vi "Process ILC Data.vi"(8 "error in (no error)":errorcluster, 11 "Model in":refnum<class "Model.lvclass">) -> (0 "error out":errorcluster, 3 "Model out":refnum<class "Model.lvclass">)   [LabVIEW 2016]
uses:
  Common_RT_FAILC/FAILC/FAILC.lvclass
  Calculators/Cylinder To Actuator Forces/Cylinder To Actuator Forces.lvclass
  Model.lvclass
  C:/CODE/ts_HPMT/Common_RT_ILC/ILC/ILC.lvclass
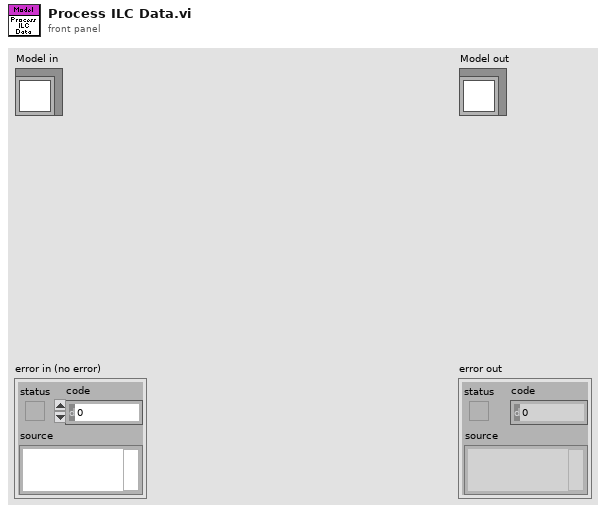
[diagram p1: front panel]
types:
  T1 = typedef "RTHPILC.lvlib/HPData.ctl" = cluster{"Constants":T2, "Command":T3, "Telemetry":T4, "Responses":T5, "Timings":T7}
  T2 = typedef "RTHPILC.lvlib/HPConstants.ctl" = cluster{"ID":i16}
  T3 = typedef "RTHPILC.lvlib/HPCommand.ctl" = cluster{"AxialSetPoint":i32, "LateralSetPoint":i32, "AxialBoosterValveGain":sgl, "LateralBoosterValveGain":sgl}
  T4 = typedef "RTHPILC.lvlib/HPTelemetry.ctl" = cluster{"ILCFault":bool, "BroadcastCounter":u8, "AxialLoadCellForce":sgl, "LateralLoadCellForce":sgl, "AxialBoosterValveGain":sgl, "LateralBoosterValveGain":sgl}
  T5 = typedef "RTHPILC.lvlib/HPResponses.ctl" = cluster{"BoosterValveGain":T6, "ReadBoosterValveGain":T6, "SetForce":T6, "ForceAndStatus":T6}
  T6 = typedef "RTModbus.lvlib/ExceptionCodes.ctl" = u16
  T7 = typedef "RTHPILC.lvlib/HPTimings.ctl" = cluster{"BroadcastSetForce":u32, "BoosterValveGain":u32, "FreezeSensorValues":u32, "ForceAndStatus":u32, "ReadBoosterValveGain":u32, "SetForce":u32}
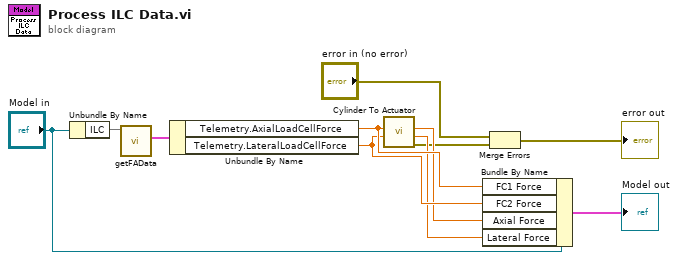
[diagram p0: block diagram]
diagram:
  n1 = Unbundle By Name("Model in") -> ("ILC"=w10)
  n2 = call "getFAData.vi"("FAILC in"=w10) -> ("FAData"=w11:T1)  [unwired: 9 in, 1 out]
  n3 = Unbundle By Name(w11) -> ("Telemetry.AxialLoadCellForce"=w8:sgl, "Telemetry.LateralLoadCellForce"=w7:sgl)
  n4 = call "Cylinder To Actuator.vi"("FC2 Measured Value"=w7, "FC1 Measured Value"=w8) -> ("error out"=w4:errorcluster, "Lateral Force"=w5:dbl, "Axial Force"=w6:dbl)  [unwired: 6 in, 1 out]
  n5 = Bundle By Name(cluster="Model in", "FC1 Force"=w8, "FC2 Force"=w7, "Axial Force"=w6, "Lateral Force"=w5) -> (→"Model out":cluster{})
  n6 = Merge Errors("error in (no error)", w4) -> (→"error out":errorcluster)
